vi "FindSimilarDataFrom2DListCtrl.vi"(9 "column index":u16, 10 "search string":string, 11 "ArrayRef in":refnum<vi>) -> (1 "is empty?":bool, 2 "array out":string[][](array[string]), 3 "ArrayRef out":refnum<vi>)   [LabVIEW 2018, in "Library-Ctrl.lvlib"]
uses:
  Library-Ctrl.lvlib
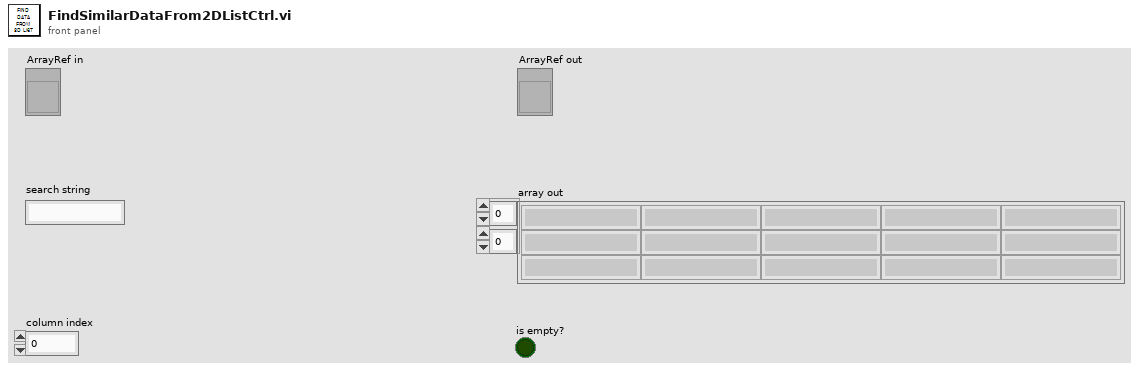
[diagram p1: front panel]
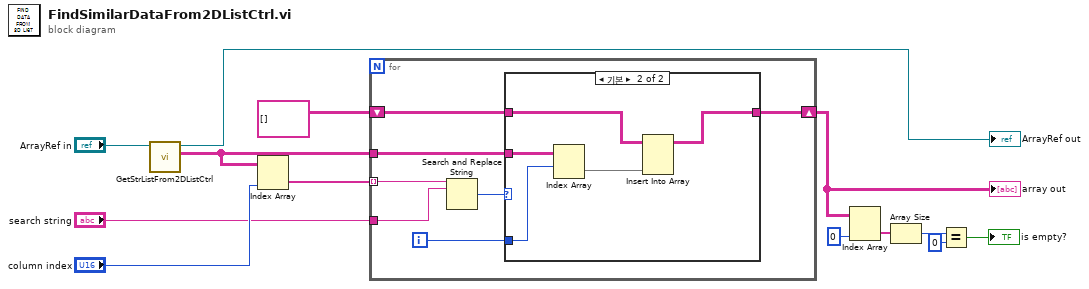
[diagram p0: block diagram]
diagram:
  n1 = call "GetStrListFrom2DListCtrl.vi"("ref 2D list in"="ArrayRef in") -> ("result"=w8:string[][], "ref 2D list out"=→"ArrayRef out":refnum<vi>)  [unwired: 9 in]
  n2 = Index Array(array=w8, index (col)="column index") -> (element=w1:string[])  [unwired: 1 in]
  n3 = for {
    tunnel: "search string" -> [w16]
    shift-right: [w19] -> w7
    shift-left: string[][] [] ("result") -> [w20]
    tunnel: w8 -> [w18]
    tunnel: w1 -> [w17] mode=indexing
    i -> [w14]
    n4 = Search and Replace String(input string=w17, search string=w16) -> (number of replacements=w15:i32)  [unwired: 6 in, 3 out]
    n5 = case shown="기본" w15 {
      tunnel: w20 -> [w21 w26]
      tunnel: [w21 w25] -> w19
      tunnel: w18 -> [_ w24]
      tunnel: w14 -> [_ w22]
      frame 0 {
      }
      frame Default {
        n6 = Index Array(array=w24, index (row)=w22) -> (element=w23:string[])  [unwired: 1 in]
        n7 = Insert Into Array(array=w26, new element=w23) -> (w25:string[][])  [unwired: 2 in]
      }
    }
  }
  "array out" <- w7
  n8 = Index Array(array=w7, index (col)=0 ("비활성화된 인덱스 (열)")) -> (element=w5:string[])  [unwired: 1 in]
  n9 = Array Size(array=w5) -> (size(s)=w4:i32)
  n10 = Equal?(x=w4, y=0) -> (x = y?=→"is empty?":bool)
